vi "create control.vi"(8 "error in":errorcluster, 9 "Create Constant":bool, 10 "terminal index":i32, 11 "object id":string) -> (0 "error out":errorcluster, 3 "new id":string)   [LabVIEW 2020]
doc: "Creates a Control, Indicator or Constant on an objects (GObject/Node) in- or output terminal. Use get_object_terminals to get the index of the terminals. Set Create Constant to true to create a constant. Otherwise will create control/indicator based on if the terminal is input or output. Returns a reference to the newly created object."
uses:
  G-AI Core/G-AI Core.lvlib
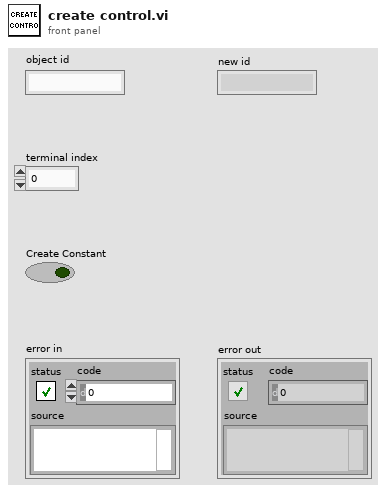
[diagram p1: front panel]
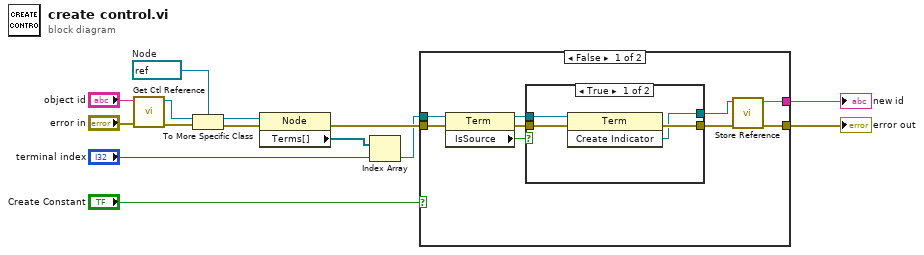
[diagram p0: block diagram]
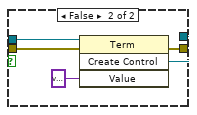
[diagram p2: hidden frame]
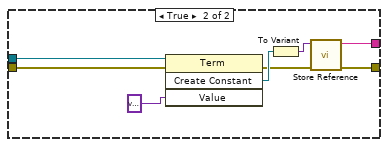
[diagram p3: hidden frame]
diagram:
  w11 = refnum<vi> refnum  # Node
  n1 = call "Get Ctl Reference.vi"("error in"="error in", "id"="object id") -> ("error out"=w13:errorcluster, "ctl reference"=w12:refnum<vi>)  [unwired: 8 in]
  n2 = To More Specific Class(target class=w11, reference=w12, error in=w13) -> (specific class reference=w8:refnum<vi>, error out=w10:errorcluster)
  n3 = property class="Node"(reference=w8, error in=w10) -> (error out=w9:errorcluster, "Terms[]"=w7:refnum<vi>[])  [unwired: 1 out]
  n4 = Index Array(array=w7, index="terminal index") -> (element=w6:refnum<vi>)
  n5 = case shown="False" "Create Constant" {
    tunnel: w9 -> [w23 w36]
    tunnel: [w17 w37] -> w2
    tunnel: w6 -> [w21 w35]
    tunnel: [w15 w34] -> w3
    frame False {
      n6 = property class="Term"(reference=w21, error in=w23) -> (reference out=w20:refnum<vi>, error out=w22:errorcluster, "IsSource"=w19:bool)
      n7 = case shown="True" w19 {
        tunnel: [w27 w32] -> w18
        tunnel: w22 -> [w26 w31]
        tunnel: w20 -> [w25 w30]
        tunnel: [w24 w29] -> w16
        frame True {
          n8 = invoke class="Term" method="Create Indicator"(reference=w25, error in=w26) -> (error out=w27:errorcluster, "Create Indicator"=w24:refnum<vi>)  [unwired: 1 in, 1 out]
        }
        frame False {
          n9 = invoke class="Term" method="Create Control"(reference=w30, error in=w31, "Value"=variant) -> (error out=w32:errorcluster, "Create Control"=w29:refnum<vi>)  [unwired: 1 in, 2 out]
        }
      }
      n10 = call "Store Reference.vi"("error in"=w18, "Reference"=w16) -> ("error out"=w17:errorcluster, "id"=w15:string)  [unwired: 8 in]
    }
    frame True {
      n11 = invoke class="Term" method="Create Constant"(reference=w35, error in=w36, "Value"=variant) -> (error out=w38:errorcluster, "Create Constant"=w40:refnum<vi>)  [unwired: 1 in, 2 out]
      n12 = To Variant(anything=w40) -> (Variant=w39:variant)
      n13 = call "Store Reference.vi"("error in"=w38, "Reference"=w39) -> ("error out"=w37:errorcluster, "id"=w34:string)  [unwired: 8 in]
    }
  }
  "new id" <- w3
  "error out" <- w2
